vi "sql-writeinfo-fixture.vi"(0 "input-IP":string="dg-sql-01.luxshare.com.cn", 1 "input-user":string="htpsuser", 2 "input-psw":string="htps'songyy", 3 "input-db":string="HTPSDB", 4 "操作模式":enum16{"写入数据", "更改数据"}(ring), 6 "表名":string="vfixture", 7 "列名":string[](array[string])=["LuxsharePN", "CustomerPN", "Customer", "ProjectName", "SampleDes", "AWG", "Length", "LimitSpec", "SwitchMatrix", "EEPROMWrite", "EEPROMContent", "LabelPrint", "LabelContent", "Remarks"], 9 "值":string[](array[string]), 11 "设置":string, 13 "条件":string) -> (12 "简单报错":string, 15 "status":bool)   [LabVIEW 2011]
panel:
  out "具体错误":string
  out "字符串":string
  out "错误输出 2":errorcluster caption="错误输出"
  out "code":i32
  out "错误输出":errorcluster
  in  "ADODB._Recordset":refnum<k7>
  in  "ADODB._Connection":refnum<k7>
  # "输       入"
  # "输       出"
  # "写入数据，需要指定写入列的名称，以及与之对应的值"
  # "基本信息\n（）"
  # "状态灯，False表示操作成功，True表示操作失败"
  # "错误信息"
  # "改变操作时需要修改的信息"
  # "操作模式：写入数据\n                  更改数据"
  # "表名"
  # "更改数据，需要指定修改列的新值"
  # "更改数据，利用条件找到需要修改的行"
  # "error:\n-2147217843 登陆失败： 。\n-2147467259 要访问的数据库不存在\n-2146825267 没有数据    。\n-2146824584 对象关闭时，不允许操作\n-2147217865 表名不存在 。\n-2147467259 服务器连接失败 。\n-2147217900 列名无效\n-2147217900 不允许有NULL值\n-2147217900 unique的键重复"
  # "error:\n-2147217900 所创建的表已经存在\n-2147217900 该列不存在"
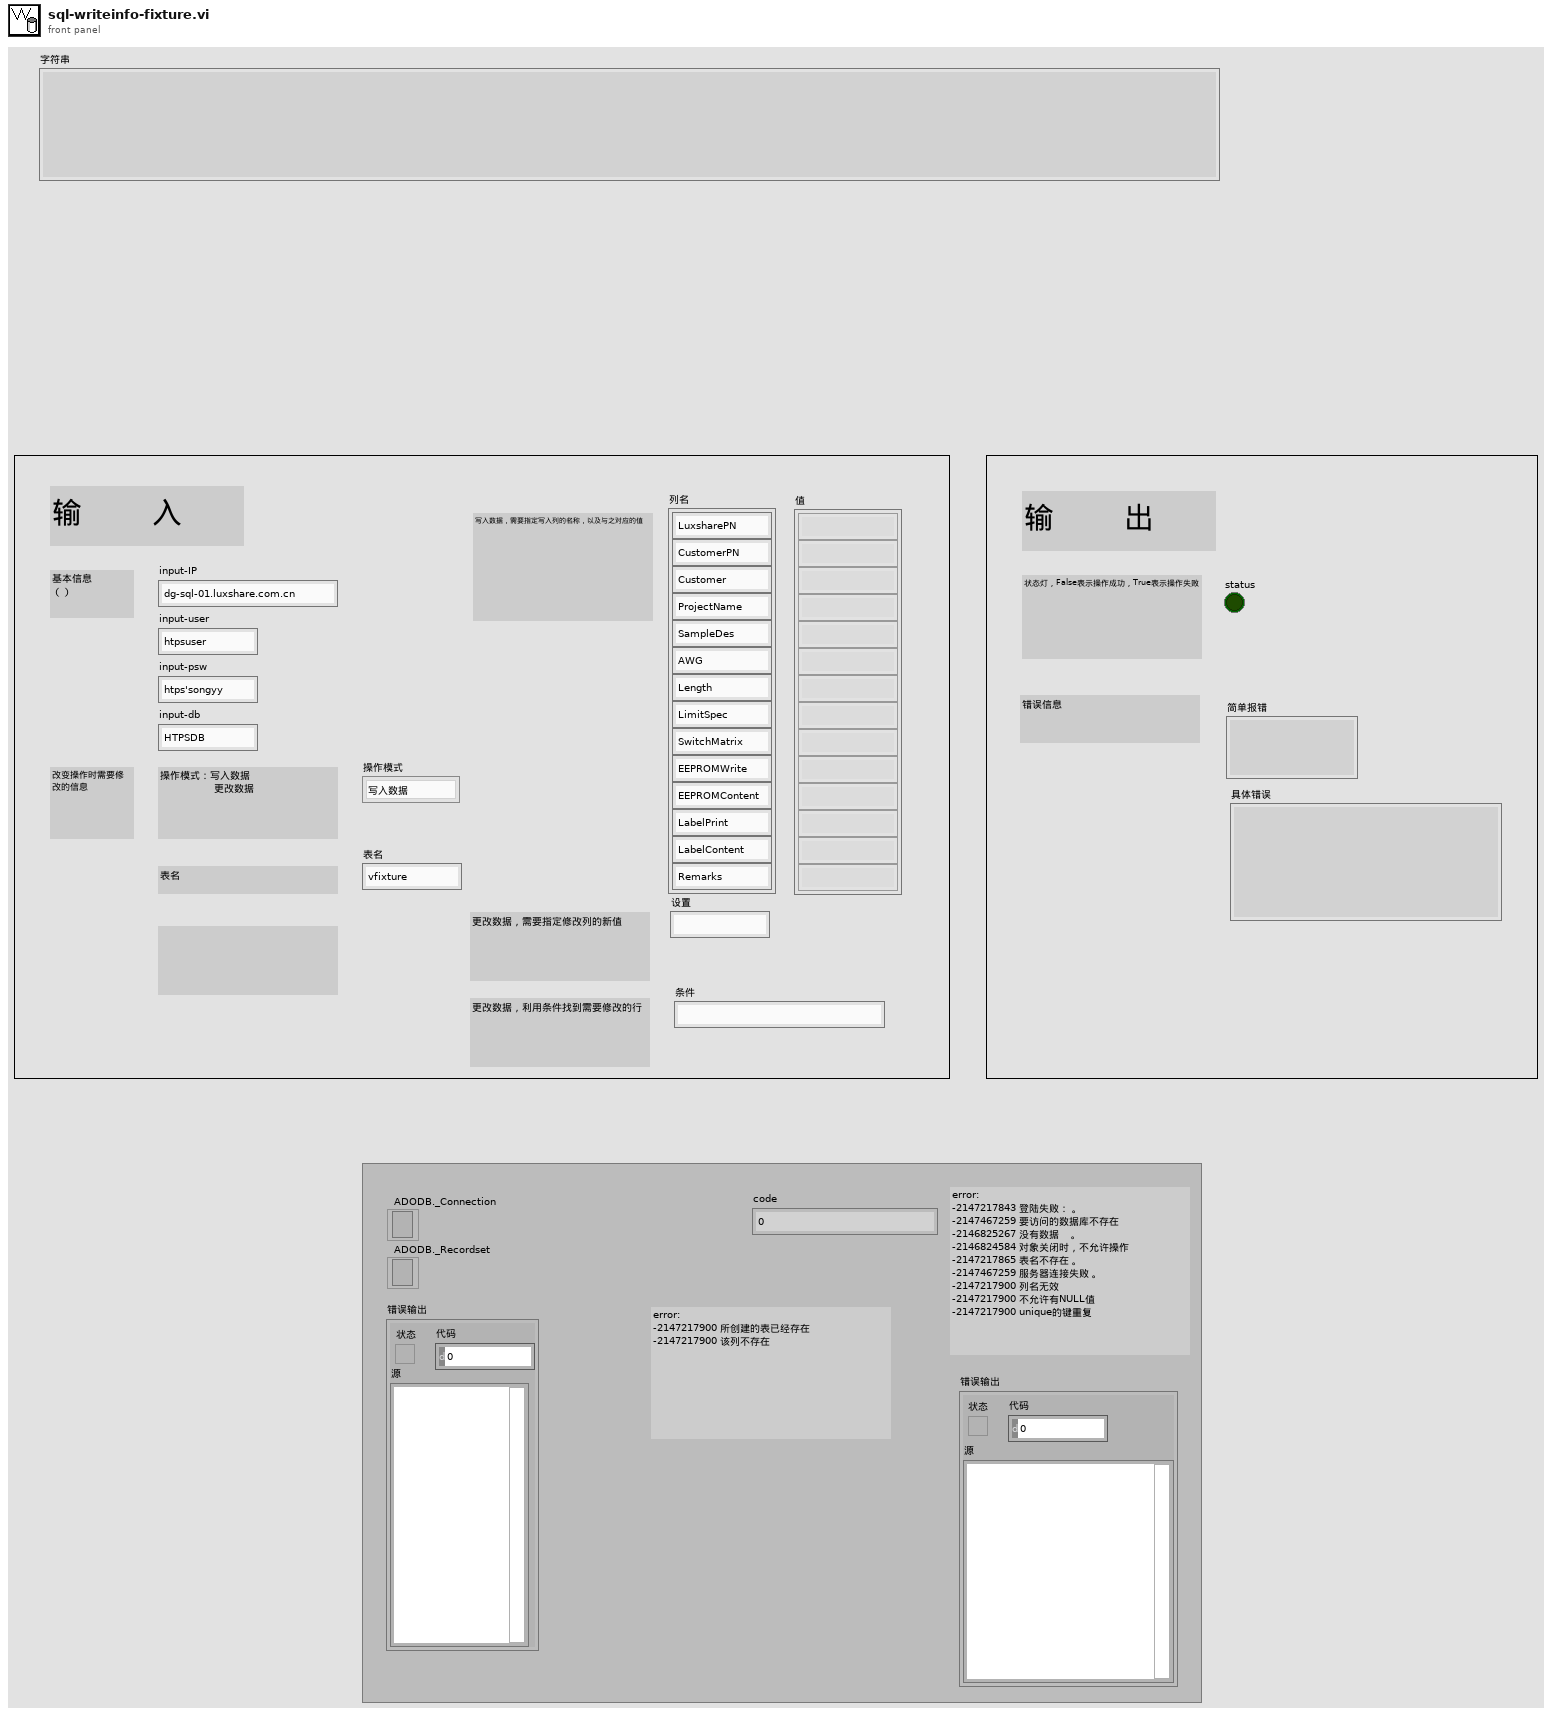
[diagram p1: front panel]
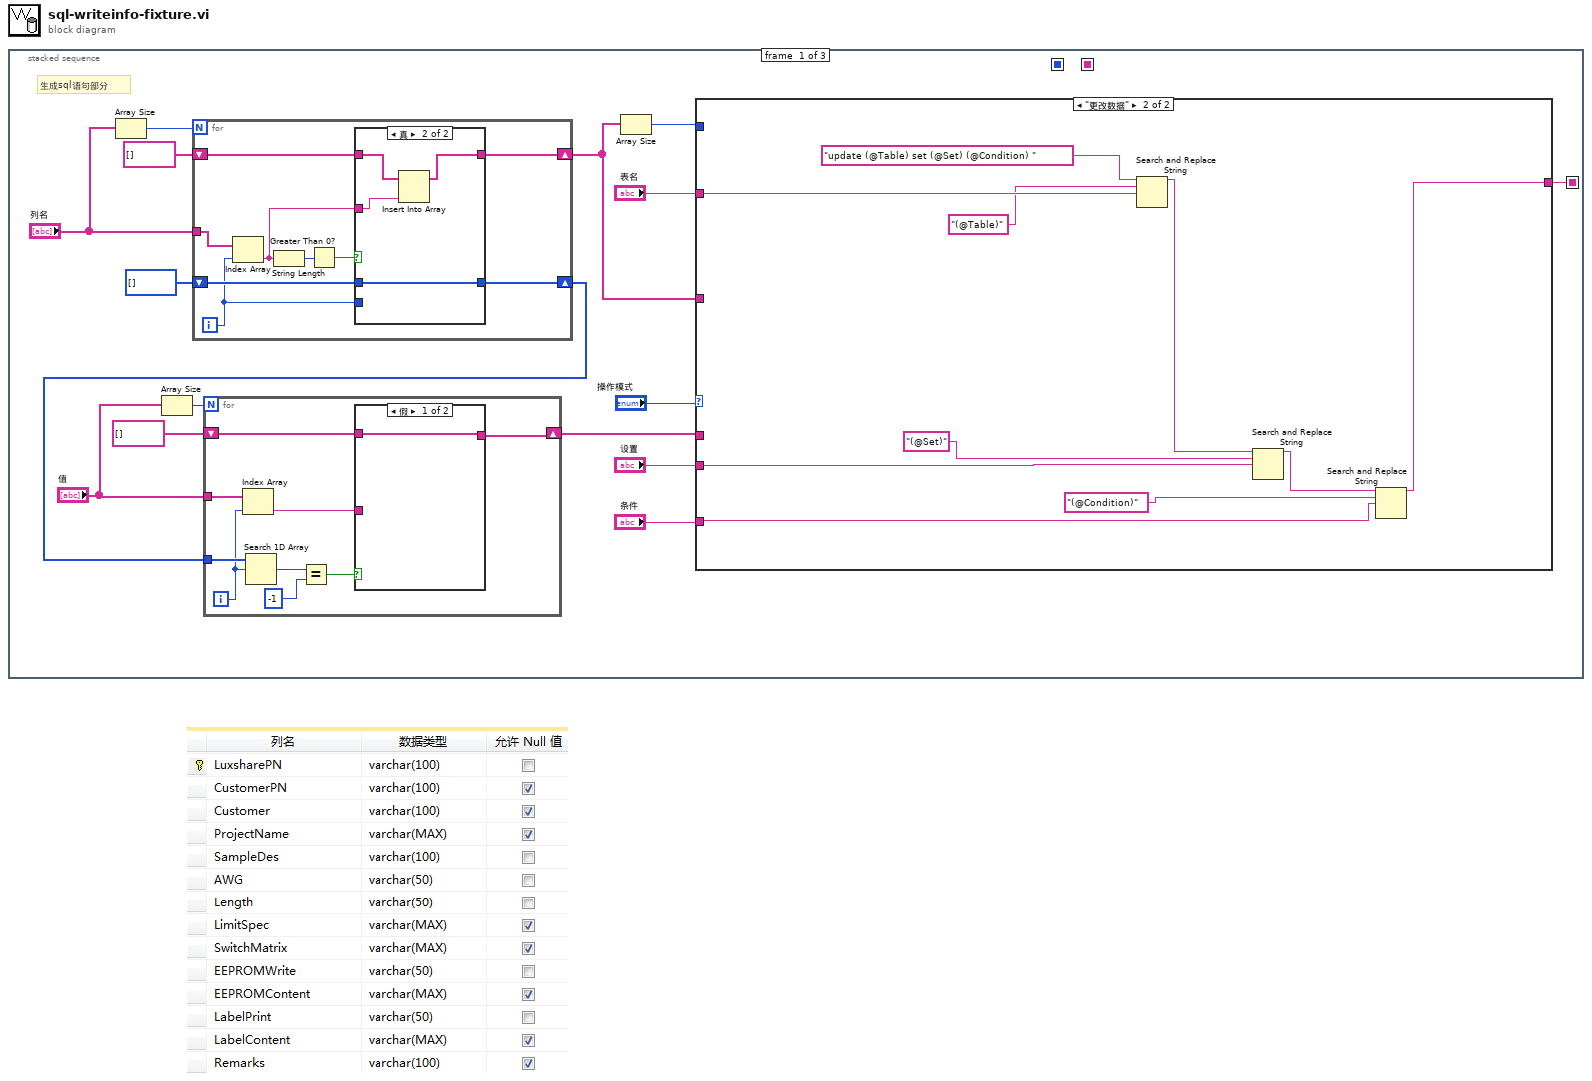
[diagram p0: block diagram]
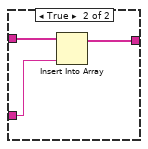
[diagram p2: hidden frame]
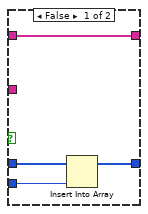
[diagram p3: hidden frame]
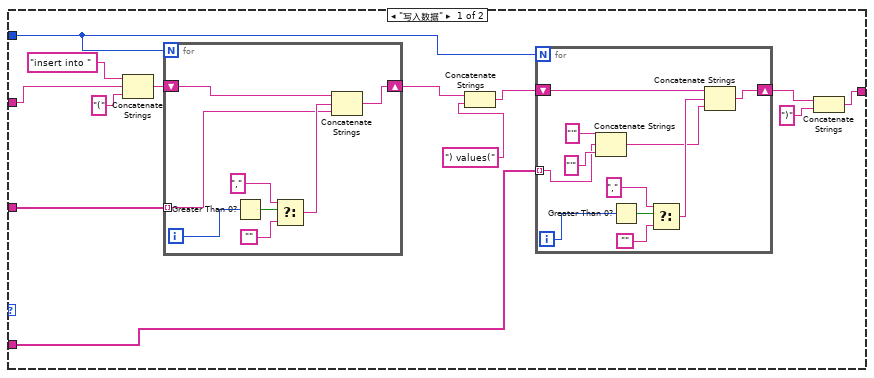
[diagram p4: hidden frame]
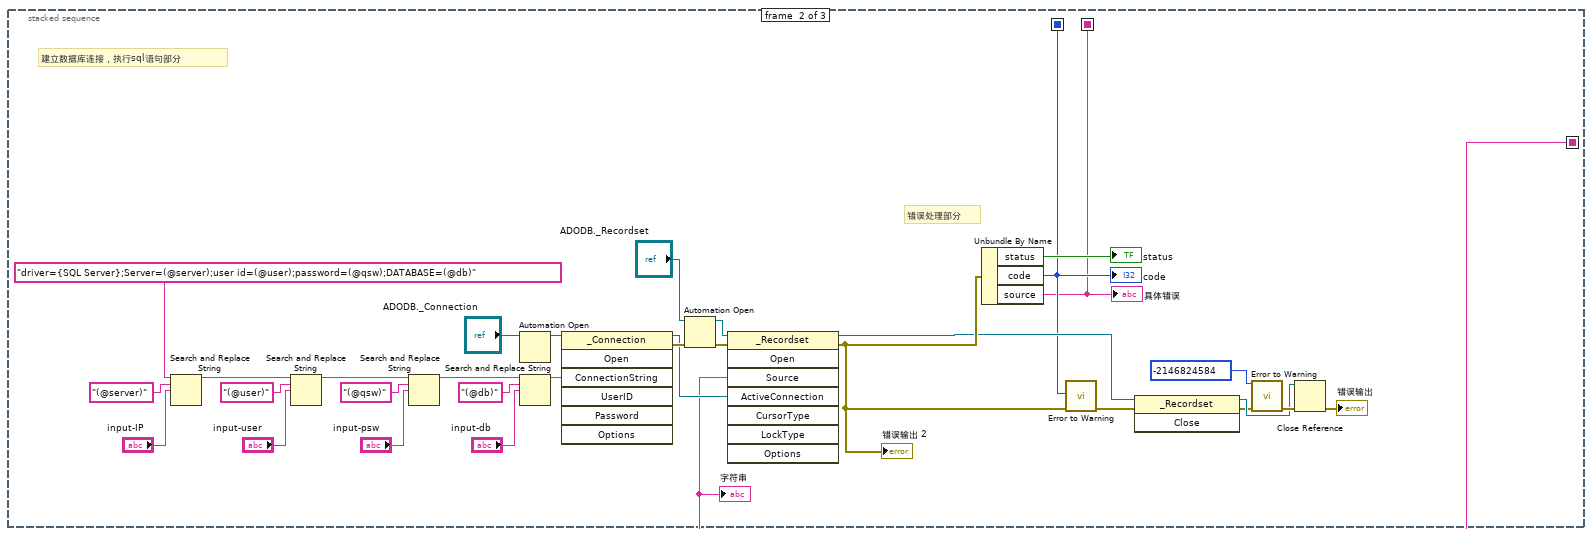
[diagram p5: hidden frame]
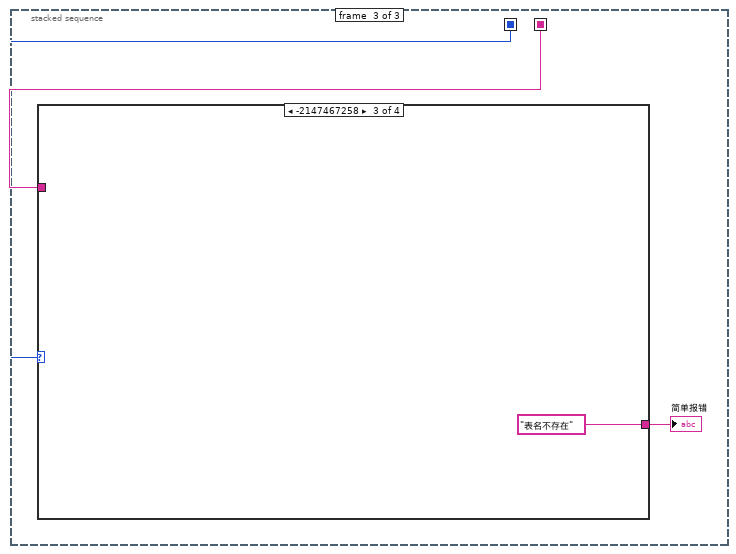
[diagram p6: hidden frame]
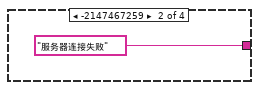
[diagram p8: hidden frame]
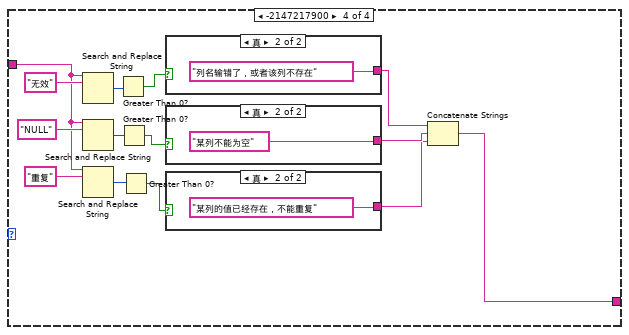
[diagram p9: hidden frame]
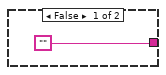
[diagram p10: hidden frame]
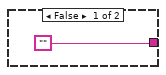
[diagram p11: hidden frame]
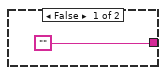
[diagram p12: hidden frame]
diagram:
  n1 = stacked-sequence {
    seq-local: [w1 _ _] -> [_ w92 _]
    seq-local: [_ w90 _] -> [_ _ w122]
    seq-local: [_ w89 _] -> [_ _ w121]
    frame #0 {
      # "生成sql语句部分"
      n2 = Array Size(array="列名") -> (size(s)=w13:i32)
      n3 = Array Size(array="值") -> (size(s)=w10:i32)
      n4 = for {
        N: w13 -> [_]
        tunnel: "列名" -> [w38]
        shift-right: [w33] -> w5
        shift-left: string[] [] -> [w34]
        shift-right: [w30] -> w8
        shift-left: i32[] [] -> [w32]
        i -> [w31]
        n5 = Index Array(array=w38, index=w31) -> (element=w35:string)
        n6 = String Length(string=w35) -> (length=w37:i32)
        n7 = Greater Than 0?(x=w37) -> (x > 0?=w36:bool)
        n8 = case shown="真" w36 {
          tunnel: w35 -> [_ w44]
          tunnel: w34 -> [w42 w46]
          tunnel: [w42 w45] -> w33
          tunnel: w32 -> [w41 w43]
          tunnel: w31 -> [w40 _]
          tunnel: [w39 w43] -> w30
          frame False {
            n9 = Insert Into Array(array=w41, new element=w40) -> (w39:i32[])  [unwired: 1 in]
          }
          frame True {
            n10 = Insert Into Array(array=w46, new element=w44) -> (w45:string[])  [unwired: 1 in]
          }
        }
      }
      n11 = for {
        N: w10 -> [_]
        shift-right: [w17] -> w4
        shift-left: string[] [] -> [w18]
        tunnel: "值" -> [w22]
        tunnel: w8 -> [w25]
        i -> [w21]
        n12 = Index Array(array=w22, index=w21) -> (element=w19:string)
        n13 = Search 1D Array(1D array=w25, element=w21) -> (index of element=w24:i32)  [unwired: 1 in]
        n14 = Equal?(x=w24, y=-1) -> (x = y?=w20:bool)
        n15 = case shown="假" w20 {
          tunnel: w19 -> [_ w27]
          tunnel: w18 -> [w26 w29]
          tunnel: [w26 w28] -> w17
          frame False {
          }
          frame True {
            n16 = Insert Into Array(array=w29, new element=w27) -> (w28:string[])  [unwired: 1 in]
          }
        }
      }
      n17 = Array Size(array=w5) -> (size(s)=w14:i32)
      n18 = case shown="\"更改数据\"" "操作模式" {
        tunnel: "表名" -> [w59 w86]
        tunnel: [w50 w79] -> w1
        tunnel: w14 -> [w56 _]
        tunnel: w5 -> [w47 _]
        tunnel: w4 -> [w49 _]
        tunnel: "设置" -> [_ w88]
        tunnel: "条件" -> [_ w80]
        frame "写入数据" {
          n19 = Concatenate Strings("insert into ", w59, "(") -> (w57:string)
          n20 = for {
            N: w56 -> [_]
            shift-right: [w72] -> w55
            shift-left: w57 -> [w78]
            tunnel: w47 -> [w73] mode=indexing
            i -> [w71]
            n21 = Greater Than 0?(x=w71) -> (x > 0?=w77:bool)
            n22 = Select(t=",", s=w77, f="") -> (s? t:f=w74:string)
            n23 = Concatenate Strings(w78, w74, w73) -> (w72:string)
          }
          n24 = Concatenate Strings(w55, ") values(") -> (w53:string)
          n25 = for {
            N: w56 -> [_]
            shift-right: [w64] -> w52
            shift-left: w53 -> [w70]
            tunnel: w49 -> [w61] mode=indexing
            i -> [w69]
            n26 = Concatenate Strings("'", w61, "'") -> (w60:string)
            n27 = Greater Than 0?(x=w69) -> (x > 0?=w68:bool)
            n28 = Select(t=",", s=w68, f="") -> (s? t:f=w65:string)
            n29 = Concatenate Strings(w70, w65, w60) -> (w64:string)
          }
          n30 = Concatenate Strings(w52, ")") -> (w50:string)
        }
        frame "更改数据" {
          n31 = Search and Replace String(input string="update (@Table) set (@Set) (@Condition) ", search string="(@Table)", replace string=w86) -> (result string=w83:string)  [unwired: 5 in, 3 out]
          n32 = Search and Replace String(input string=w83, search string="(@Set)", replace string=w88) -> (result string=w82:string)  [unwired: 5 in, 3 out]
          n33 = Search and Replace String(input string=w82, search string="(@Condition)", replace string=w80) -> (result string=w79:string)  [unwired: 5 in, 3 out]
        }
      }
    }
    frame #1 {
      # "错误处理部分"
      # "建立数据库连接，执行sql语句部分"
      n34 = Search and Replace String(input string="driver={SQL Server};Server=(@server);user id=(@user);password=(@qsw);DATABASE=(@db)" ("ConnectionString"), search string="(@server)" ("搜索字符串"), replace string="input-IP") -> (result string=w97:string)  [unwired: 5 in, 3 out]
      n35 = Search and Replace String(input string=w97, search string="(@user)" ("搜索字符串"), replace string="input-user") -> (result string=w100:string)  [unwired: 5 in, 3 out]
      n36 = Search and Replace String(input string=w100, search string="(@qsw)" ("搜索字符串"), replace string="input-psw") -> (result string=w103:string)  [unwired: 5 in, 3 out]
      n37 = Automation Open(Automation Refnum="ADODB._Connection") -> (Automation Refnum=w93:refnum<k7>)  [unwired: 3 in, 1 out]
      n38 = Search and Replace String(input string=w103, search string="(@db)" ("搜索字符串"), replace string="input-db") -> (result string=w107:string)  [unwired: 5 in, 3 out]
      n39 = invoke class="_Connection" method="Open"(reference=w93, "ConnectionString"=w107) -> (reference out=w109:refnum<k7>, error out=w111:errorcluster)  [unwired: 5 in, 5 out]
      n40 = Automation Open(error in (no error)=w111, Automation Refnum="ADODB._Recordset") -> (Automation Refnum=w110:refnum<k7>, error out=w112:errorcluster)  [unwired: 2 in]
      n41 = invoke class="_Recordset" method="Open"(reference=w110, error in=w112, "Source"=w92, "ActiveConnection"=w109) -> (reference out=w119:refnum<k7>, error out=w120:errorcluster)  [unwired: 4 in, 6 out]
      "错误输出 2" <- w120
      n42 = Unbundle By Name(w120) -> ("status"=→"status":bool, "code"=w90:i32, "source"=w89:string)
      "code" <- w90
      "具体错误" <- w89
      n43 = call <vilib>:"Error to Warning.vi"("1st Error to Convert"=w90, "error in"=w120) -> ("warning out"=w113:errorcluster)  [unwired: 13 in]
      n44 = invoke class="_Recordset" method="Close"(reference=w119, error in=w113) -> (reference out=w117:refnum<k7>, error out=w114:errorcluster)  [unwired: 1 in, 1 out]
      n45 = call <vilib>:"Error to Warning.vi"("1st Error to Convert"=-2146824584, "error in"=w114) -> ("warning out"=w118:errorcluster)  [unwired: 13 in]
      n46 = Close Reference(reference=w117, error in (no error)=w118) -> (error out=→"错误输出":errorcluster)
      "字符串" <- w92
    }
    frame #2 {
      n47 = case shown="-2147467258" w122 {
        tunnel: [_ "服务器连接失败" "表名不存在" w126] -> w123
        tunnel: w121 -> [_ _ _ w137]
        frame 0, Default {
        }
        frame -2147467259 {
        }
        frame -2147467258 {
        }
        frame -2147217900 {
          n48 = Search and Replace String(input string=w137, search string="无效" ("搜索字符串")) -> (number of replacements=w135:i32)  [unwired: 6 in, 3 out]
          n49 = Search and Replace String(input string=w137, search string="NULL" ("搜索字符串")) -> (number of replacements=w134:i32)  [unwired: 6 in, 3 out]
          n50 = Search and Replace String(input string=w137, search string="重复" ("搜索字符串")) -> (number of replacements=w133:i32)  [unwired: 6 in, 3 out]
          n51 = Greater Than 0?(x=w135) -> (x > 0?=w132:bool)
          n52 = Greater Than 0?(x=w134) -> (x > 0?=w131:bool)
          n53 = Greater Than 0?(x=w133) -> (x > 0?=w130:bool)
          n54 = case shown="真" w132 {
            tunnel: ["" "列名输错了，或者该列不存在"] -> w129
            frame False {
            }
            frame True {
            }
          }
          n55 = case shown="真" w131 {
            tunnel: ["" "某列不能为空"] -> w128
            frame False {
            }
            frame True {
            }
          }
          n56 = case shown="真" w130 {
            tunnel: ["" "某列的值已经存在，不能重复"] -> w127
            frame False {
            }
            frame True {
            }
          }
          n57 = Concatenate Strings(w129, w128, w127) -> (w126:string)
        }
      }
      "简单报错" <- w123
    }
  }
